vi "robot main.vi"() -> ()   [LabVIEW 2011]
doc: "This VI imlements the framework and scheduler for your robotics program. It should not be necessary to modify the framework. You are expected to add your code to the VIs called from Robot Main, the ones located in the Team Code within the project."
uses:
  <vilib>/Rock Robotics/WPI/Camera/WPI_CameraImageSize.ctl
  <vilib>/Rock Robotics/WPI/SafetyOutput/WPI_SafetyOutputConfigMenu.ctl
  Robot Global Data.vi
panel:
  out "Lag Millis":u32
  in  "Image Size":T1=enum."320x240"
  in  "Finish":bool
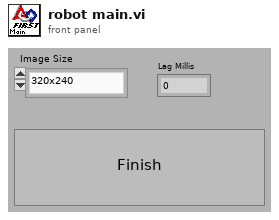
[diagram p1: front panel]
types:
  T1 = typedef "WPI_CameraImageSize.ctl" = enum16{"640x480", "320x240", "160x120"}
  T2 = typedef "WPI_DriverStationMatch Info.ctl" = cluster{"Autonomous Elapsed Seconds":dbl, "TeleOp Elapsed Seconds":dbl, "Disabled Elapsed Seconds":dbl, "Visited Autonomous":bool, "Visited TeleOp":bool, "Visited Disabled":bool, "Autonomous Settings":cluster{"Autonomous Style":enum16{"Iterative", "Independent"}, "VI Refnum":refnum<vi>}}
  T3 = typedef "WPI_DriverStationDerivedRobotMode.ctl" = enum16{"Init", "Execute", "Stop"}
  T4 = typedef "WPI_DriverStationRobotMode.ctl" = enum16{"Autonomous Disabled", "Autonomous Enabled", "Teleop Disabled", "Teleop Enabled", "Timeout", "Finish"}
  T5 = typedef "WPI_SafetyOutputConfigMenu.ctl" = enum16{"Enable", "Disable"}
  T6 = typedef "WPI_MotorControlDeviceRef.ctl" = cluster{"DeviceStatus":errorcluster, "Type":enum16{"PWM", "CAN"}, "PWM":cluster{"Digital Module":T7, "PWM Channel":T8, "DeadBand":T9}, "CAN":cluster{"Device Number":u8, "Control Mode":T10, "Semaphore":T11, "Max Vout":dbl}, "Invert":bool, "TransformRef":T12, "InvTransformRef":T12}
  T7 = typedef "FPGA_TypedefDigitalModule.ctl" = enum16{"Digital Module 1", "Digital Module 2"}
  T8 = typedef "FPGA_DIOPWMChannel.ctl" = enum8{"PWM 1", "PWM 2", "PWM 3", "PWM 4", "PWM 5", "PWM 6", "PWM 7", "PWM 8", "PWM 9", "PWM 10", "Invalid"}
  T9 = typedef "WPI_PWMDeadband.ctl" = cluster{"Name":string, "maxPositivePwm":i32, "minPositivePwm":i32, "centerPwm":i32, "maxNegativePwm":i32, "minNegativePwm":i32, "angularRange":u16}
  T10 = typedef "WPI_CANJaguar_ControlMode.ctl" = enum8{"Percent VBus", "Current", "Speed", "Position", "Voltage"}
  T11 = typedef "Semaphore RefNum" = refnum<k1>
  T12 = typedef "WPI_PWMTransform_ConPane.ctl" = refnum<vi>
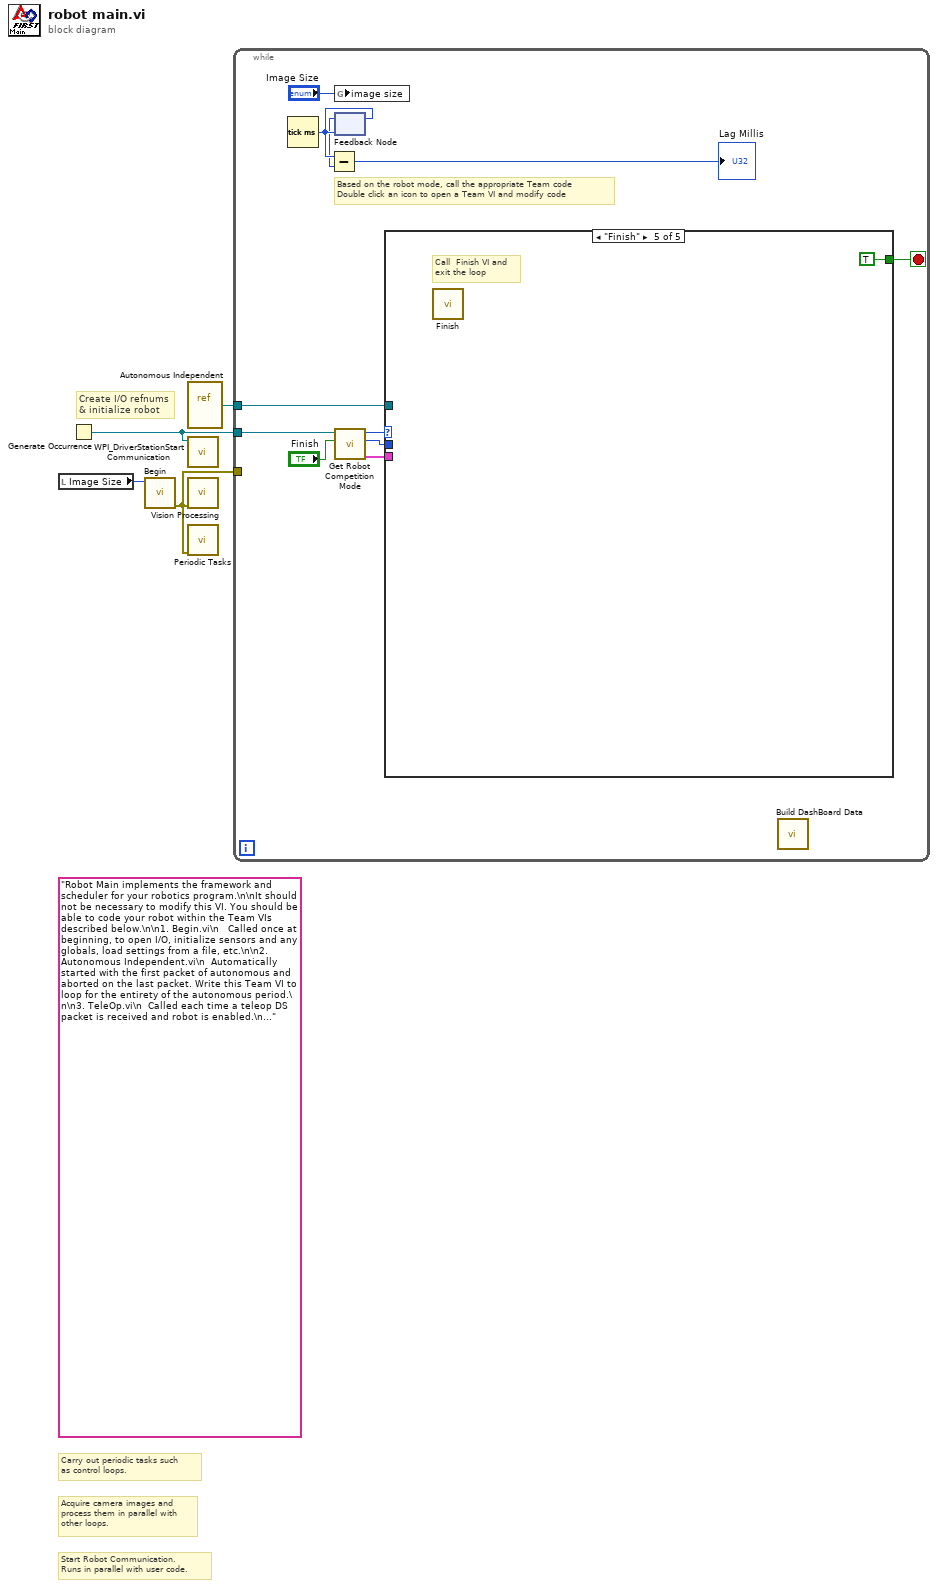
[diagram p0: block diagram]
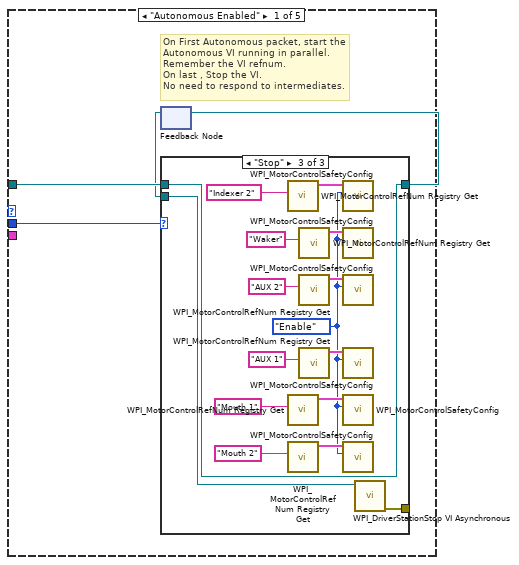
[diagram p2: hidden frame]
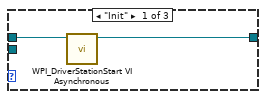
[diagram p3: hidden frame]
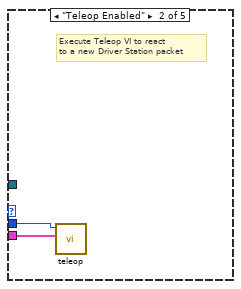
[diagram p5: hidden frame]
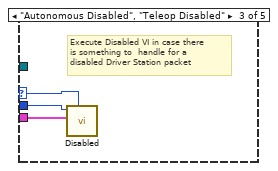
[diagram p6: hidden frame]
diagram:
  (unwired) "Robot Main implements the framework and scheduler for your robotics program.\n\nIt should not be necessary to modify this VI. You should be able to code your robot within the Team VIs described below.\n\n1. Begin.vi\n   Called once at beginning, to open I/O, initialize sensors and any globals, load settings from a file, etc.\n\n2. Autonomous Independent.vi\n  Automatically started with the first packet of autonomous and aborted on the last packet. Write this Team VI to loop for the entirety of the autonomous period.\n\n3. TeleOp.vi\n  Called each time a teleop DS packet is received and robot is enabled.\n\n4. Disabled.vi\n  Called each time a packet is received and the robot is disabled.\n\n5. Vision.vi\n  A parallel loop that acquires and processes camera images.\n\n6. PeriodicTasks.vi\n  Parallel loops running at user-defined rates.\n\n7. Finish.vi\n  Called before exiting, so you can save data, clean up I/O, etc.\n\n8. Build DashBoard Data.vi\n  Called for each driver station packet including timeouts. It is used to send select I/O values back to the Dashboard."
  # "Start Robot Communication.\nRuns in parallel with user code."
  # "Acquire camera images and\nprocess them in parallel with\nother loops."
  # "Carry out periodic tasks such\nas control loops."
  # "Create I/O refnums\n& initialize robot"
  n1 = local read "Image Size"() -> (w3:T1)
  n2 = Generate Occurrence() -> (w4:refnum<k4>)
  n3 = call "Begin.vi"("Image Size"=w3) -> ("error out"=w1:errorcluster)  [unwired: 10 out]
  n4 = vi-ref "Autonomous Independent.vi"() -> (w2:refnum<vi>)
  n5 = call <vilib>:"WPI_DriverStationStart Communication.vi"("occurrence"=w4) -> ()  [unwired: 11 out]
  n6 = call "Vision Processing.vi"("error in (no error)"=w1) -> ()  [unwired: 2 in, 5 out]
  n7 = call "Periodic Tasks.vi"("error in (no error)"=w1) -> ()  [unwired: 1 in, 10 out]
  n8 = while {
    tunnel: w4 -> [w13]
    tunnel: w1 -> [_]
    tunnel: w2 -> [w9]
    stop <- w10 stop-if-true
    # "Based on the robot mode, call the appropriate Team code\nDouble click an icon to open a Team VI and modify code"
    n9 = Tick Count (ms)() -> (millisecond timer value=w7:u32)
    n10 = global write "Robot Global Data.vi" "image size"("Image Size") -> ()
    n11 = feedback-in #1(w7) -> ()
    n12 = feedback #1(w7) -> (w6:u32)
    n13 = Subtract(x=w7, y=w6) -> (x-y=→"Lag Millis":u32)
    n14 = call "Get Robot Competition Mode.vi"("Finish"="Finish", "DS Occurrence"=w13) -> ("Match Info out"=w11:T2, "Call Context"=w15:T3, "Robot Mode"=w14:T4)  [unwired: 7 out]
    n15 = case shown="\"Finish\"" w14 {
      selector: w14 -> [_ _ w41 _ _]
      tunnel: w15 -> [w19 w40 w43 _ _]
      tunnel: w11 -> [_ w39 w42 _ _]
      tunnel: [_ _ _ _ TRUE] -> w10
      tunnel: w9 -> [w18 _ _ _ _]
      frame "Autonomous Enabled" {
        # "On First Autonomous packet, start the\nAutonomous VI running in parallel.\nRemember the VI refnum.\nOn last , Stop the VI.\nNo need to respond to intermediates."
        n16 = feedback #2() -> (w16:refnum<vi>)  [unwired: 1 out]
        n17 = case shown="\"Stop\"" w19 {
          tunnel: w18 -> [w21 _ w37]
          tunnel: [w20 w22 w37] -> w17
          tunnel: w16 -> [_ w22 w38]
          tunnel: [_ _ w36] -> _
          frame "Init" {
            n18 = call <vilib>:"WPI_DriverStationStart VI Asynchronous.vi"("VI"=w21) -> ("VI out"=w20:refnum<vi>)  [unwired: 10 out]
          }
          frame "Execute", Default {
            # "Nothing to do"
          }
          frame "Stop" {
            w23 = WPI_SafetyOutputConfigMenu."Enable" ("mode")
            n19 = call <vilib>:"WPI_MotorControlRefNum Registry Get.vi"("refnum name"="Indexer 2") -> ("MotorControlDevRef"=w33:T6)  [unwired: 9 in, 1 out]
            n20 = call <vilib>:"WPI_MotorControlRefNum Registry Get.vi"("refnum name"="Mouth 1") -> ("MotorControlDevRef"=w31:T6)  [unwired: 9 in, 1 out]
            n21 = call <vilib>:"WPI_MotorControlRefNum Registry Get.vi"("refnum name"="Mouth 2") -> ("MotorControlDevRef"=w28:T6)  [unwired: 9 in, 1 out]
            n22 = call <vilib>:"WPI_MotorControlRefNum Registry Get.vi"("refnum name"="Waker") -> ("MotorControlDevRef"=w32:T6)  [unwired: 9 in, 1 out]
            n23 = call <vilib>:"WPI_MotorControlRefNum Registry Get.vi"("refnum name"="AUX 2") -> ("MotorControlDevRef"=w24:T6)  [unwired: 9 in, 1 out]
            n24 = call <vilib>:"WPI_MotorControlRefNum Registry Get.vi"("refnum name"="AUX 1") -> ("MotorControlDevRef"=w27:T6)  [unwired: 9 in, 1 out]
            n25 = call <vilib>:"WPI_MotorControlSafetyConfig.vi"("mode"=w23, "MotorControlDevRef"=w33) -> ()  [unwired: 8 in, 2 out]
            n26 = call <vilib>:"WPI_MotorControlSafetyConfig.vi"("mode"=w23, "MotorControlDevRef"=w32) -> ()  [unwired: 8 in, 2 out]
            n27 = call <vilib>:"WPI_MotorControlSafetyConfig.vi"("mode"=w23, "MotorControlDevRef"=w24) -> ()  [unwired: 8 in, 2 out]
            n28 = call <vilib>:"WPI_MotorControlSafetyConfig.vi"("mode"=w23, "MotorControlDevRef"=w27) -> ()  [unwired: 8 in, 2 out]
            n29 = call <vilib>:"WPI_MotorControlSafetyConfig.vi"("mode"=w23, "MotorControlDevRef"=w31) -> ()  [unwired: 8 in, 2 out]
            n30 = call <vilib>:"WPI_MotorControlSafetyConfig.vi"("mode"=w23, "MotorControlDevRef"=w28) -> ()  [unwired: 8 in, 2 out]
            n31 = call <vilib>:"WPI_DriverStationStop VI Asynchronous.vi"("VI Refnum"=w38) -> ("error out"=w36:errorcluster)  [unwired: 10 out]
          }
        }
        n32 = feedback-in #2(w17) -> ()
      }
      frame "Teleop Enabled" {
        # "Execute Teleop VI to react\nto a new Driver Station packet"
        n33 = call "teleop.vi"("Match Info"=w39, "Call Context"=w40) -> ()  [unwired: 10 in]
      }
      frame "Autonomous Disabled", "Teleop Disabled" {
        # "Execute Disabled VI in case there\nis something to  handle for a\ndisabled Driver Station packet"
        n34 = call "Disabled.vi"("Robot Mode"=w41, "Match Info"=w42, "Call Context"=w43) -> ()  [unwired: 1 in, 8 out]
      }
      frame "Timeout" {
        # "Driver Station packet didn't arrive.\nPossibly useful for diagnostics"
      }
      frame "Finish" {
        # "Call  Finish VI and\nexit the loop"
        n35 = call "Finish.vi"() -> ()  [unwired: 1 in, 7 out]
      }
    }
    n36 = call "Build DashBoard Data.vi"() -> ()  [unwired: 1 in, 11 out]
  }
